vi "Induction Matrix Model.vi"(0 "Basic Cells":u64, 1 "Advanced Cells":u64, 2 "Elite Cells":u64, 3 "Ultimate Cells":u64, 4 "Basic Providers":u64, 5 "Advanced Providers":u64, 6 "Elite Providers":u64, 7 "Ultimate Providers":u64, 8 "Width (m)":u32=3 min=3 max=18 step=1, 10 "Length (m)":u32=3 min=3 max=18 step=1, 12 "Height (m)":u32=4 min=3 max=18 step=1) -> (20 "Total Blocks":u32, 21 "Fits In Structure?":bool, 22 "Volume (m³)":u32, 23 "Internal Volume (m³)":u32, 24 "Storage (GFE)":ext, 25 "Storage (FE)":u64, 26 "Provider Rate (kFE/t)":ext, 27 "Provider Rate (FE/t)":u64)   [LabVIEW 2023]
panel:
  # "Induction Matrix Build"
  # "Induction Matrix Population"
  # "8GJ\n64GJ\n512GJ\n4TJ"
  # "256kJ\n2.048MJ\n16.384MJ\n131.072MJ"
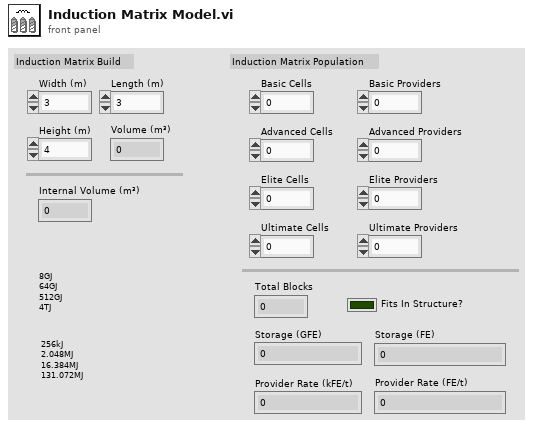
[diagram p1: front panel]
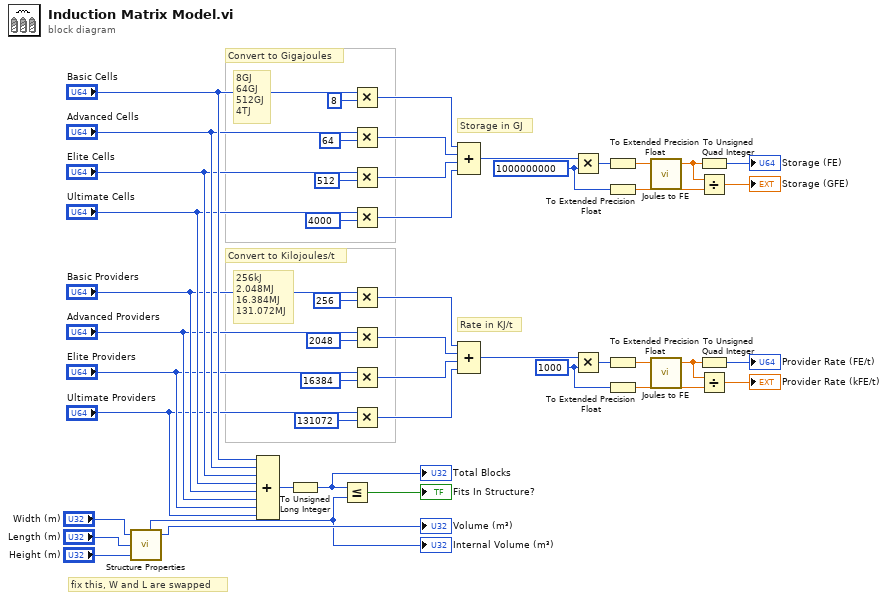
[diagram p0: block diagram]
diagram:
  w7 = u64 1000000000 ("y")
  w10 = u64 1000 ("y")
  # "fix this, W and L are swapped"
  # "Rate in KJ/t"
  # "Storage in GJ"
  # "Convert to Kilojoules/t"
  # "256kJ\n2.048MJ\n16.384MJ\n131.072MJ"
  # "8GJ\n64GJ\n512GJ\n4TJ"
  # "Convert to Gigajoules"
  n1 = call "Structure Properties.vi"("Length"="Width (m)", "Width"="Length (m)", "Height"="Height (m)") -> ("Inner Volume"=w26:i32, "Volume"=→"Volume (m³)":i32)  [unwired: 2 in, 3 out]
  "Internal Volume (m³)" <- w26
  n2 = Compound Arithmetic op=ADD("Basic Cells", "Advanced Cells", "Elite Cells", "Ultimate Cells", "Basic Providers", "Advanced Providers", "Elite Providers", "Ultimate Providers") -> (w27:u64)
  n3 = To Unsigned Long Integer(number=w27) -> (unsigned 32bit integer=w25:u32)
  "Total Blocks" <- w25
  n4 = Less Or Equal?(x=w25, y=w26) -> (x <= y?=→"Fits In Structure?":bool)
  n5 = Multiply(x="Basic Cells", y=u64 8) -> (x*y=w24:u64)
  n6 = Multiply(x="Advanced Cells", y=u64 64) -> (x*y=w23:u64)
  n7 = Multiply(x="Elite Cells", y=u64 512) -> (x*y=w21:u64)
  n8 = Multiply(x="Ultimate Cells", y=u64 4000) -> (x*y=w22:u64)
  n9 = Multiply(x="Basic Providers", y=u64 256) -> (x*y=w20:u64)
  n10 = Multiply(x="Advanced Providers", y=u64 2048) -> (x*y=w19:u64)
  n11 = Multiply(x="Elite Providers", y=u64 16384) -> (x*y=w18:u64)
  n12 = Multiply(x="Ultimate Providers", y=u64 131072) -> (x*y=w17:u64)
  n13 = Compound Arithmetic op=ADD(w24, w23, w21, w22) -> (w14:u64)
  n14 = Compound Arithmetic op=ADD(w20, w19, w18, w17) -> (w16:u64)
  n15 = Multiply(x=w14, y=w7) -> (x*y=w13:u64)
  n16 = Multiply(x=w16, y=w10) -> (x*y=w15:u64)
  n17 = To Extended Precision Float(1:w13) -> (0:w12:ext)
  n18 = To Extended Precision Float(1:w7) -> (0:w8:ext)
  n19 = To Extended Precision Float(1:w15) -> (0:w11:ext)
  n20 = To Extended Precision Float(1:w10) -> (0:w9:ext)
  n21 = call "Joules to FE.vi"("J"=w12) -> ("FE"=w4:dbl)  [unwired: 4 in]
  n22 = call "Joules to FE.vi"("J"=w11) -> ("FE"=w2:dbl)  [unwired: 4 in]
  n23 = To Unsigned Quad Integer(1:w4) -> (0:→"Storage (FE)":u64)
  n24 = Divide(x=w4, y=w8) -> (x/y=→"Storage (GFE)":ext)
  n25 = To Unsigned Quad Integer(1:w2) -> (0:→"Provider Rate (FE/t)":u64)
  n26 = Divide(x=w2, y=w9) -> (x/y=→"Provider Rate (kFE/t)":ext)
